vi "数据解析.vi"(9 "LIN数据帧数组":T1[](array[typedef])) -> (1 "LIN数据帧数组 out":T1[](array[typedef]), 4 "LIN报文显示":string[][](table))   [LabVIEW 2020, in "zlgcan.lvlib"]
uses:
  zlgcan.lvlib
  ZCAN_LIN_MSG.ctl
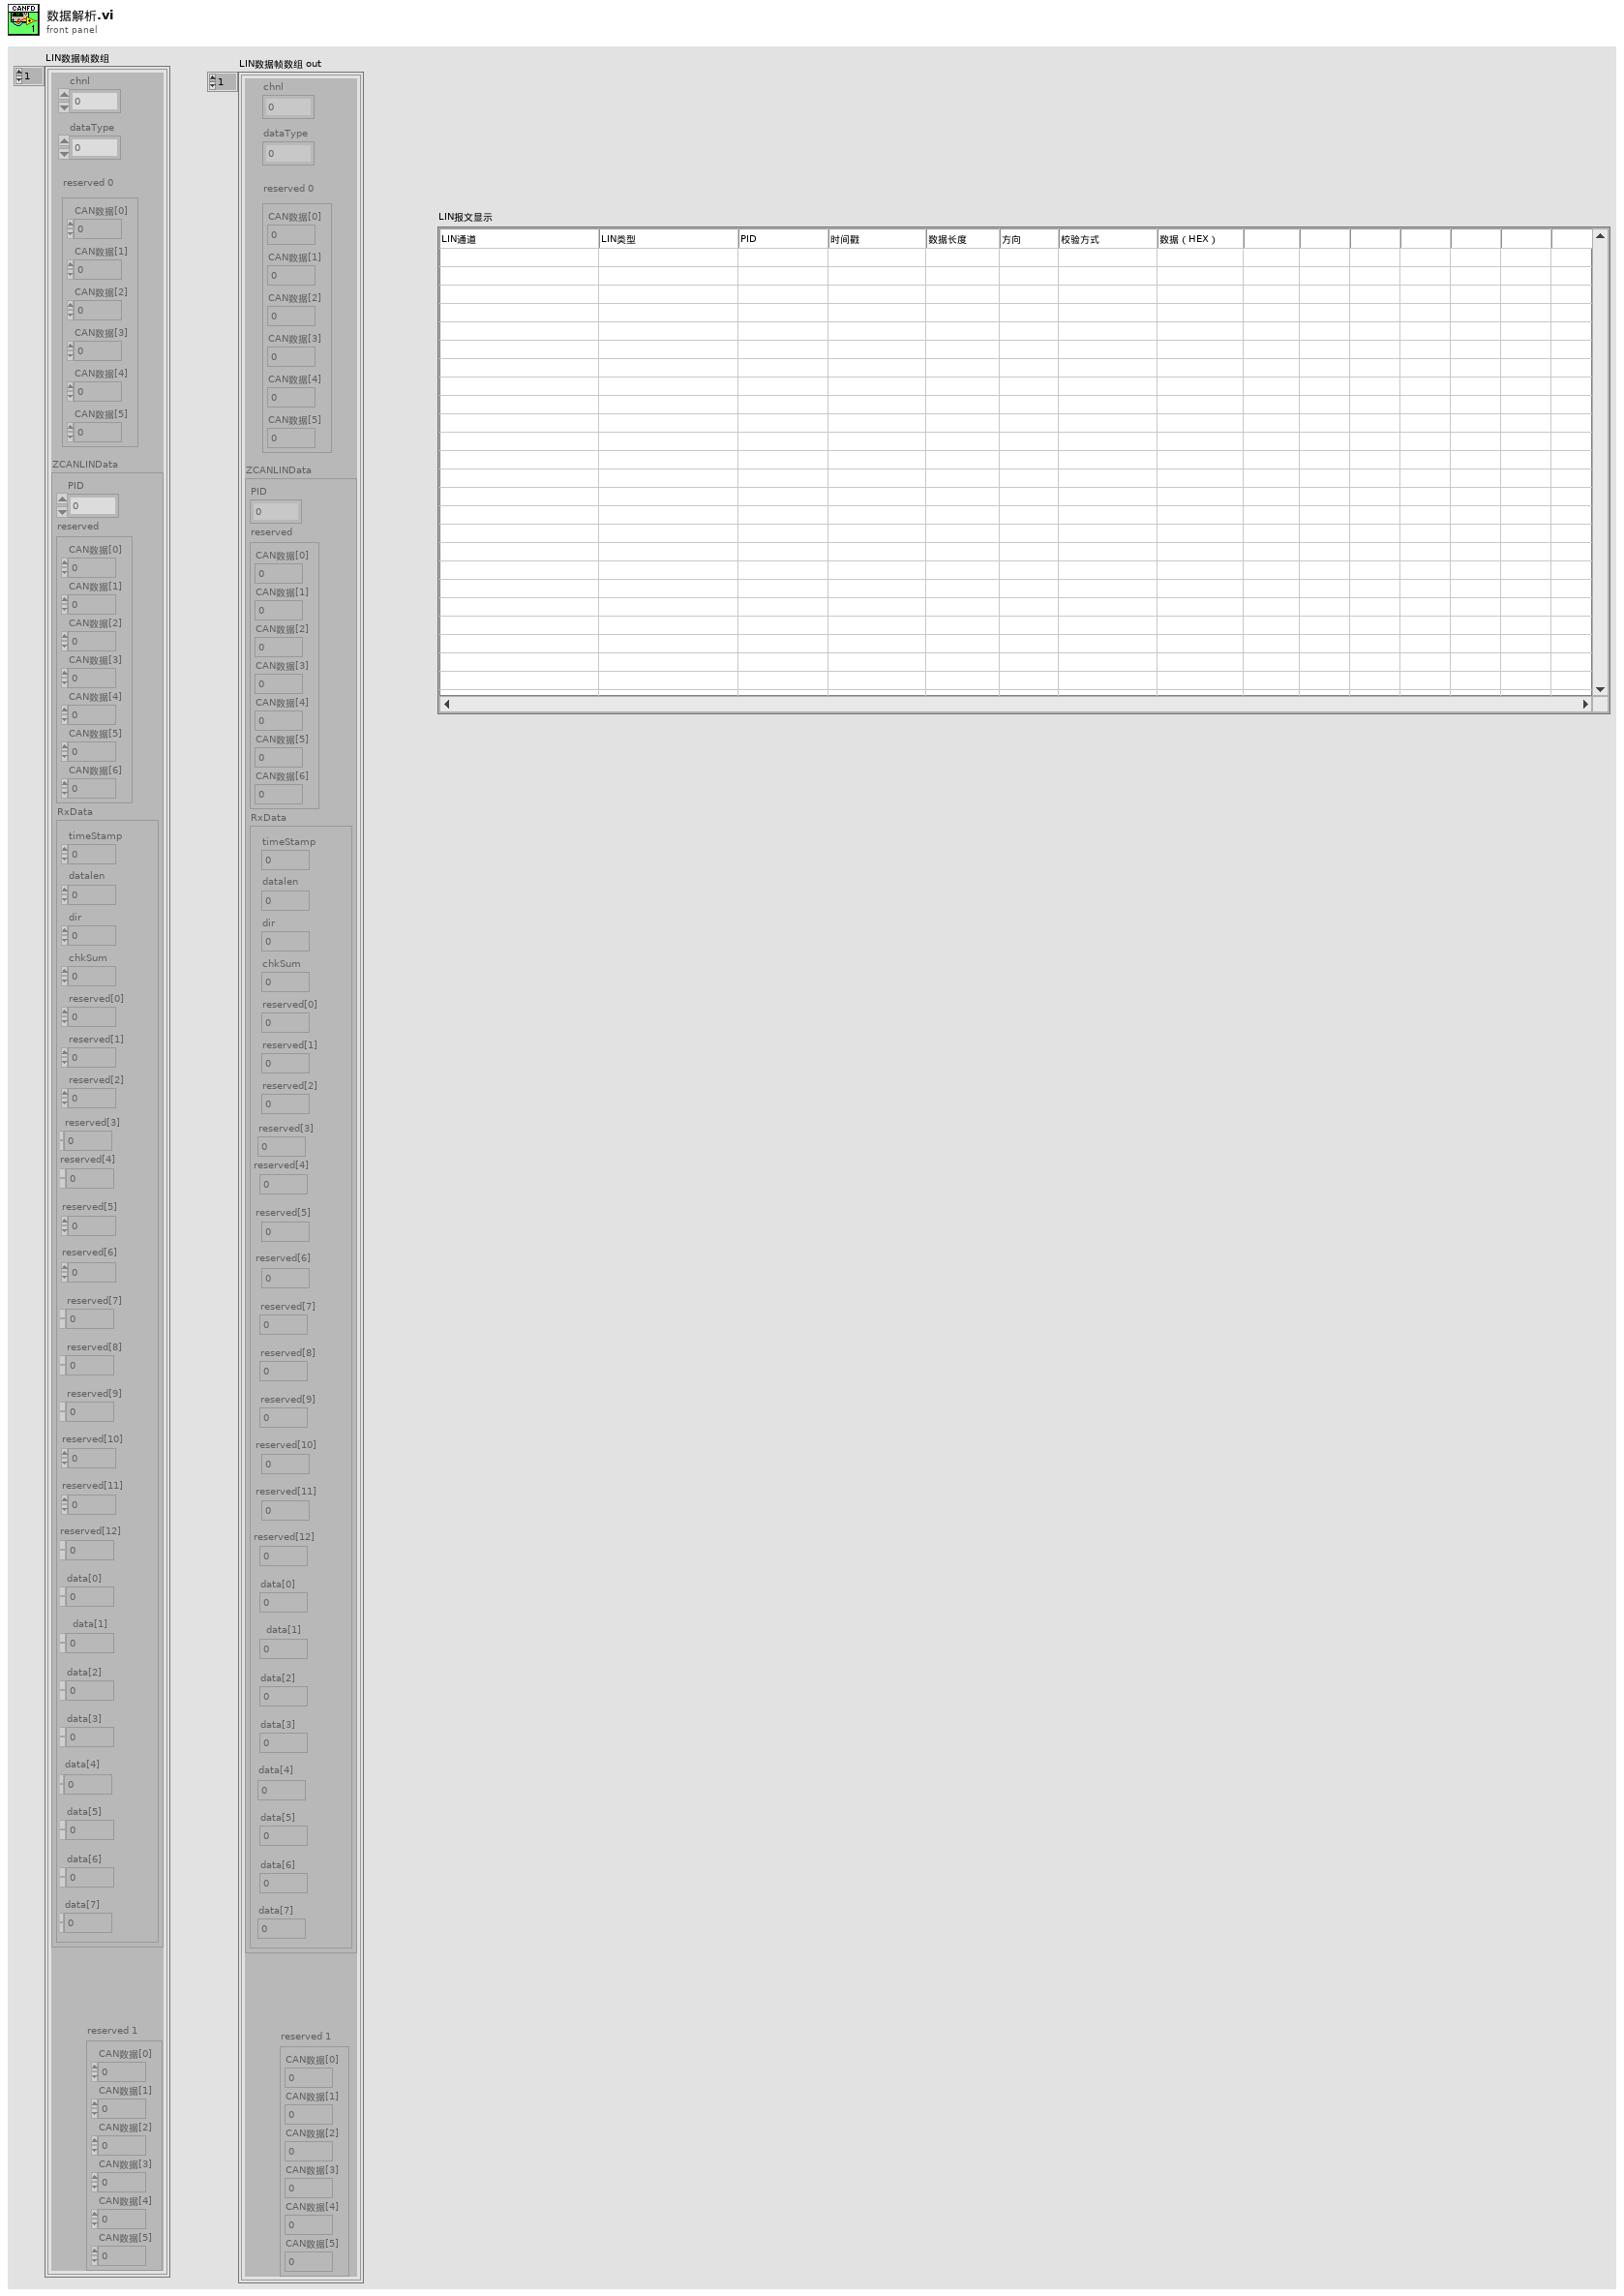
[diagram p1: front panel]
types:
  T1 = typedef "zlgcan.lvlib/ZCAN_LIN_MSG.ctl" = cluster{"chnl":u8, "dataType":u8, "reserved 0":cluster{"CAN数据[0]":u8, "CAN数据[1]":u8, "CAN数据[2]":u8, "CAN数据[3]":u8, "CAN数据[4]":u8, "CAN数据[5]":u8}, "ZCANLINData":cluster{"PID":u8, "reserved":cluster{"CAN数据[0]":u8, "CAN数据[1]":u8, "CAN数据[2]":u8, "CAN数据[3]":u8, "CAN数据[4]":u8, "CAN数据[5]":u8, "CAN数据[6]":u8}, "RxData":cluster{"timeStamp":u64, "datalen":u8, "dir":u8, "chkSum":u8, "reserved[0]":u8, "reserved[1]":u8, "reserved[2] ":u8, "reserved[3]":u8, "reserved[4]":u8, "reserved[5]":u8, "reserved[6] ":u8, "reserved[7] ":u8, "reserved[8]":u8, "reserved[9] ":u8, "reserved[10] ":u8, "reserved[11] ":u8, "reserved[12] ":u8, "data[0]":u8, "data[1]":u8, "data[2]":u8, "data[3]":u8, "data[4]":u8, "data[5]":u8, "data[6]":u8, "data[7]":u8}}, "reserved 1":cluster{"CAN数据[0]":u8, "CAN数据[1]":u8, "CAN数据[2]":u8, "CAN数据[3]":u8, "CAN数据[4]":u8, "CAN数据[5]":u8}}
  T2 = cluster{"PID":u8, "reserved":cluster{"CAN数据[0]":u8, "CAN数据[1]":u8, "CAN数据[2]":u8, "CAN数据[3]":u8, "CAN数据[4]":u8, "CAN数据[5]":u8, "CAN数据[6]":u8}, "RxData":cluster{"timeStamp":u64, "datalen":u8, "dir":u8, "chkSum":u8, "reserved[0]":u8, "reserved[1]":u8, "reserved[2] ":u8, "reserved[3]":u8, "reserved[4]":u8, "reserved[5]":u8, "reserved[6] ":u8, "reserved[7] ":u8, "reserved[8]":u8, "reserved[9] ":u8, "reserved[10] ":u8, "reserved[11] ":u8, "reserved[12] ":u8, "data[0]":u8, "data[1]":u8, "data[2]":u8, "data[3]":u8, "data[4]":u8, "data[5]":u8, "data[6]":u8, "data[7]":u8}}
  T3 = cluster{"timeStamp":u64, "datalen":u8, "dir":u8, "chkSum":u8, "reserved[0]":u8, "reserved[1]":u8, "reserved[2] ":u8, "reserved[3]":u8, "reserved[4]":u8, "reserved[5]":u8, "reserved[6] ":u8, "reserved[7] ":u8, "reserved[8]":u8, "reserved[9] ":u8, "reserved[10] ":u8, "reserved[11] ":u8, "reserved[12] ":u8, "data[0]":u8, "data[1]":u8, "data[2]":u8, "data[3]":u8, "data[4]":u8, "data[5]":u8, "data[6]":u8, "data[7]":u8}
  T4 = cluster{"data[0]":u8, "data[1]":u8, "data[2]":u8, "data[3]":u8, "data[4]":u8, "data[5]":u8, "data[6]":u8, "data[7]":u8}
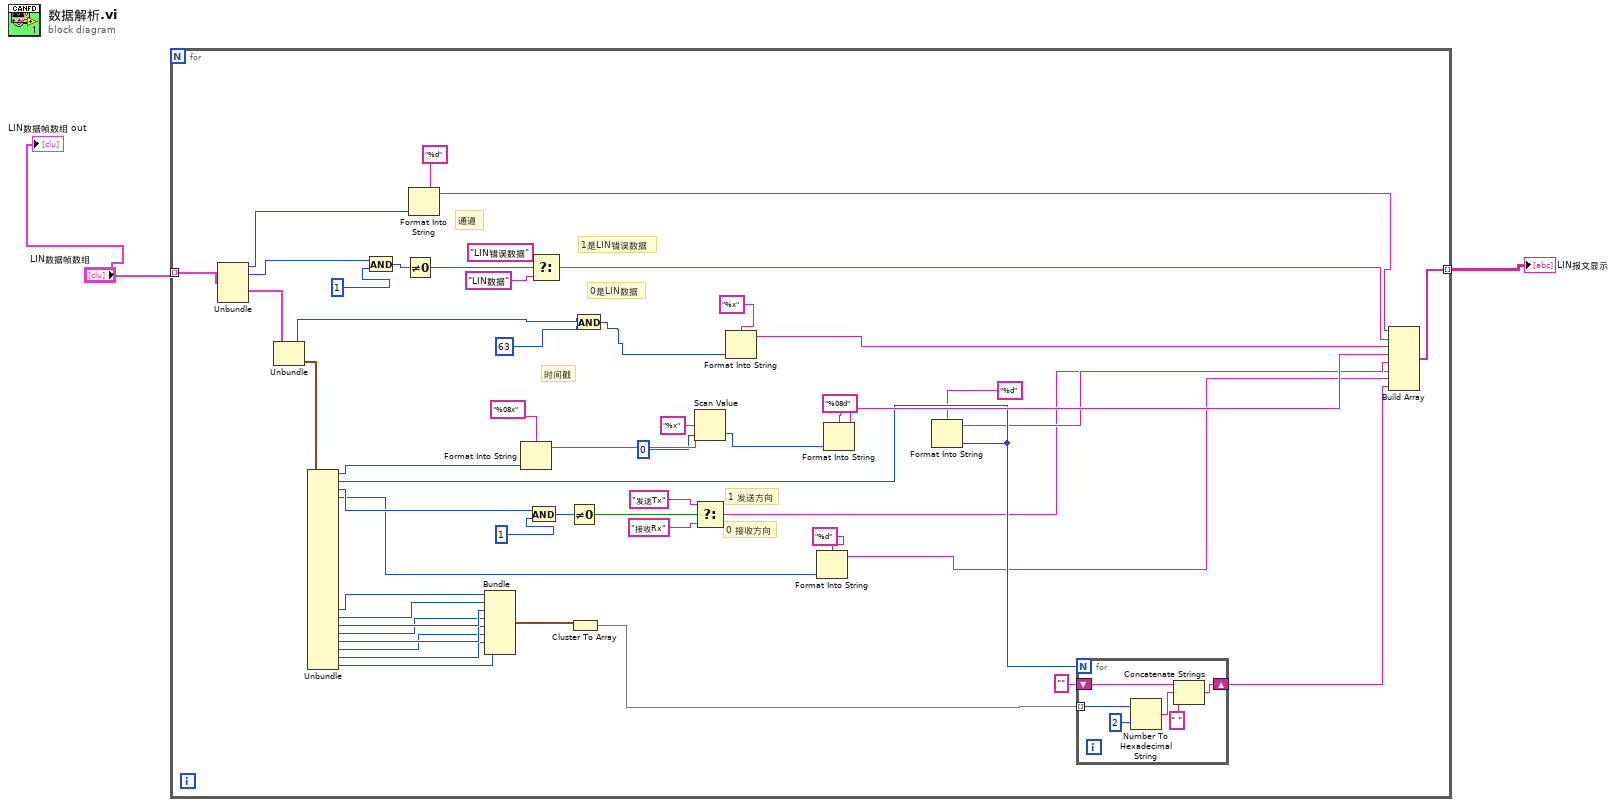
[diagram p0: block diagram]
diagram:
  n1 = for {
    tunnel: [w54] -> w1 mode=indexing
    tunnel: "LIN数据帧数组" -> [w5] mode=indexing
    # "0 接收方向"
    # "1 发送方向"
    # "1是LIN错误数据"
    # "0是LIN数据"
    # "时间戳"
    # "通道"
    n2 = Unbundle(w5) -> ("chnl"=w41:u8, "dataType"=w28:u8, "ZCANLINData"=w4:T2)  [unwired: 2 out]
    n3 = Unbundle(w4) -> ("PID"=w8:u8, "RxData"=w3:T3)  [unwired: 1 out]
    n4 = Unbundle(w3) -> ("timeStamp"=w34:u64, "datalen"=w26:u8, "dir"=w18:u8, "chkSum"=w11:u8, "data[0]"=w52:u8, "data[1]"=w51:u8, "data[2]"=w50:u8, "data[3]"=w49:u8, "data[4]"=w48:u8, "data[5]"=w47:u8, "data[6]"=w46:u8, "data[7]"=w45:u8)  [unwired: 13 out]
    n5 = And(x=w28, y=u32 1) -> (x .and. y?=w32:u32)
    n6 = Not Equal To 0?(x=w32) -> (x != 0?=w29:bool)
    n7 = Format Into String(format string="%d", w41) -> (resulting string=w16:string)  [unwired: 2 in, 1 out]
    n8 = Bundle("data[0]"=w52, "data[1]"=w51, "data[2]"=w50, "data[3]"=w49, "data[4]"=w48, "data[5]"=w47, "data[6]"=w46, "data[7]"=w45) -> (w44:T4)  [unwired: 1 in]
    n9 = Format Into String(format string="%08x", w34) -> (resulting string=w39:string)  [unwired: 2 in, 1 out]
    n10 = And(x=w18, y=u32 1) -> (x .and. y?=w23:u32)
    n11 = Select(t="LIN错误数据", s=w29, f="LIN数据") -> (s? t:f=w15:string)
    n12 = Not Equal To 0?(x=w23) -> (x != 0?=w20:bool)
    n13 = Cluster To Array(cluster=w44) -> (array=w43:u8[])
    n14 = And(x=w8, y=u8 63) -> (x .and. y?=w6:u8)
    n15 = Scan Value(string=w39, format string="%x", default (0 dbl)=0) -> (value=w35:i32)  [unwired: 1 out]
    n16 = Select(t="发送Tx", s=w20, f="接收Rx") -> (s? t:f=w17:string)
    n17 = Format Into String(format string="%x", w6) -> (resulting string=w12:string)  [unwired: 2 in, 1 out]
    n18 = Format Into String(format string="%d", w11) -> (resulting string=w10:string)  [unwired: 2 in, 1 out]
    n19 = Format Into String(format string="%08d", w35) -> (resulting string=w33:string)  [unwired: 2 in, 1 out]
    n20 = Format Into String(format string="%d", w26) -> (resulting string=w24:string)  [unwired: 2 in, 1 out]
    n21 = for {
      N: w26 -> [_]
      shift-right: [w57] -> w25
      shift-left: "" -> [w55]
      tunnel: w43 -> [w56] mode=indexing
      n22 = Number To Hexadecimal String(1:i16 2 ("width (-)"), 2:w56) -> (0:w59:string)
      n23 = Concatenate Strings(w55, w59, " " ("string")) -> (w57:string)
    }
    n24 = Build Array(w16, w15, w12, w33, w24, w17, w10, w25) -> (w54:string[])
  }
  "LIN报文显示" <- w1
  "LIN数据帧数组 out" <- "LIN数据帧数组"
